vi "testRx.vi"() -> ()   [LabVIEW 2013]
uses:
  lv_lib/CHR34XXX.lvlib
panel:
  in  "通道号":u8 max=23 step=1
  out "devId":i32
  in  "Mode":u8
  in  "pstRsdcb":T1
  out "Exit":bool
  in  "退出":bool
  out "RxFlag":bool
  in  "开始接收":bool
  out "RxData(Hex)":string
  out "布尔":bool
  in  "通道号":u8 max=23 step=1
  # "Mode：通道模式，0 表示 232 模式，1 表示 422 模式，2 表示 485 模式 \nBaudRate：波特率\nRS232：75~500Kbps\nRS422/485：75~2.4Mbps\nByteSize：数据位长度，取值范围为 5~8\nStopBits：停止位个数，取值范围为 0~2\n取值为 0 时，表示 1 位停止位(ByteSize 取值为 5~8)\n取值为 1 时，表示 1.5 位停止位(ByteSize 取值为 5)\n取值为 2 时，表示 2 位停止位(ByteSize 取值为 6~8)\nParity：校验方式，取值范围为 0~4\n0：无校验，1：奇校验，2：偶校验，3：Mark 校验，4：Space 校验"
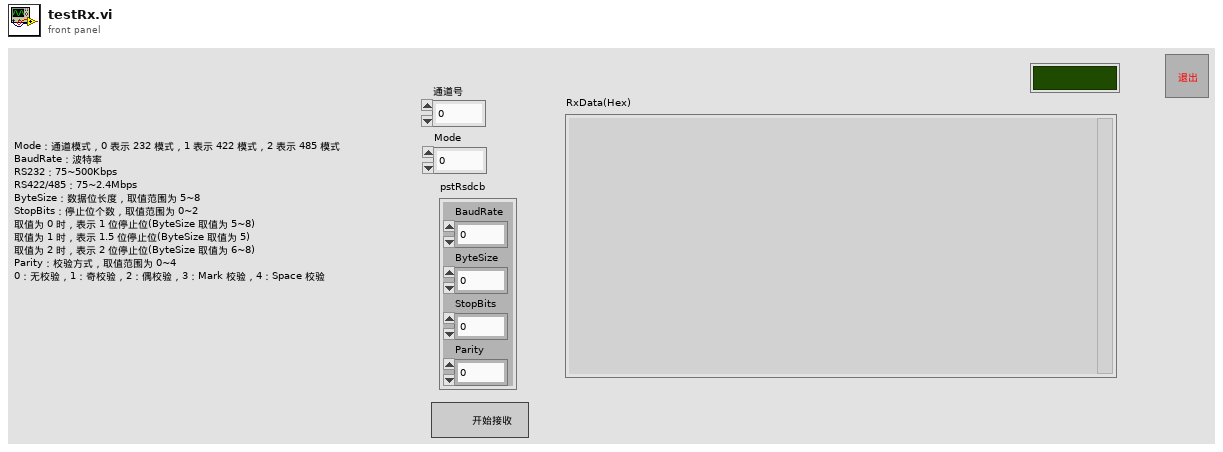
[diagram p1: front panel]
types:
  T1 = cluster{"BaudRate":u32, "ByteSize":u32, "StopBits":u32, "Parity":u32}
  T2 = enum8{"Enabled", "Disabled", "Disabled and Grayed Out"}
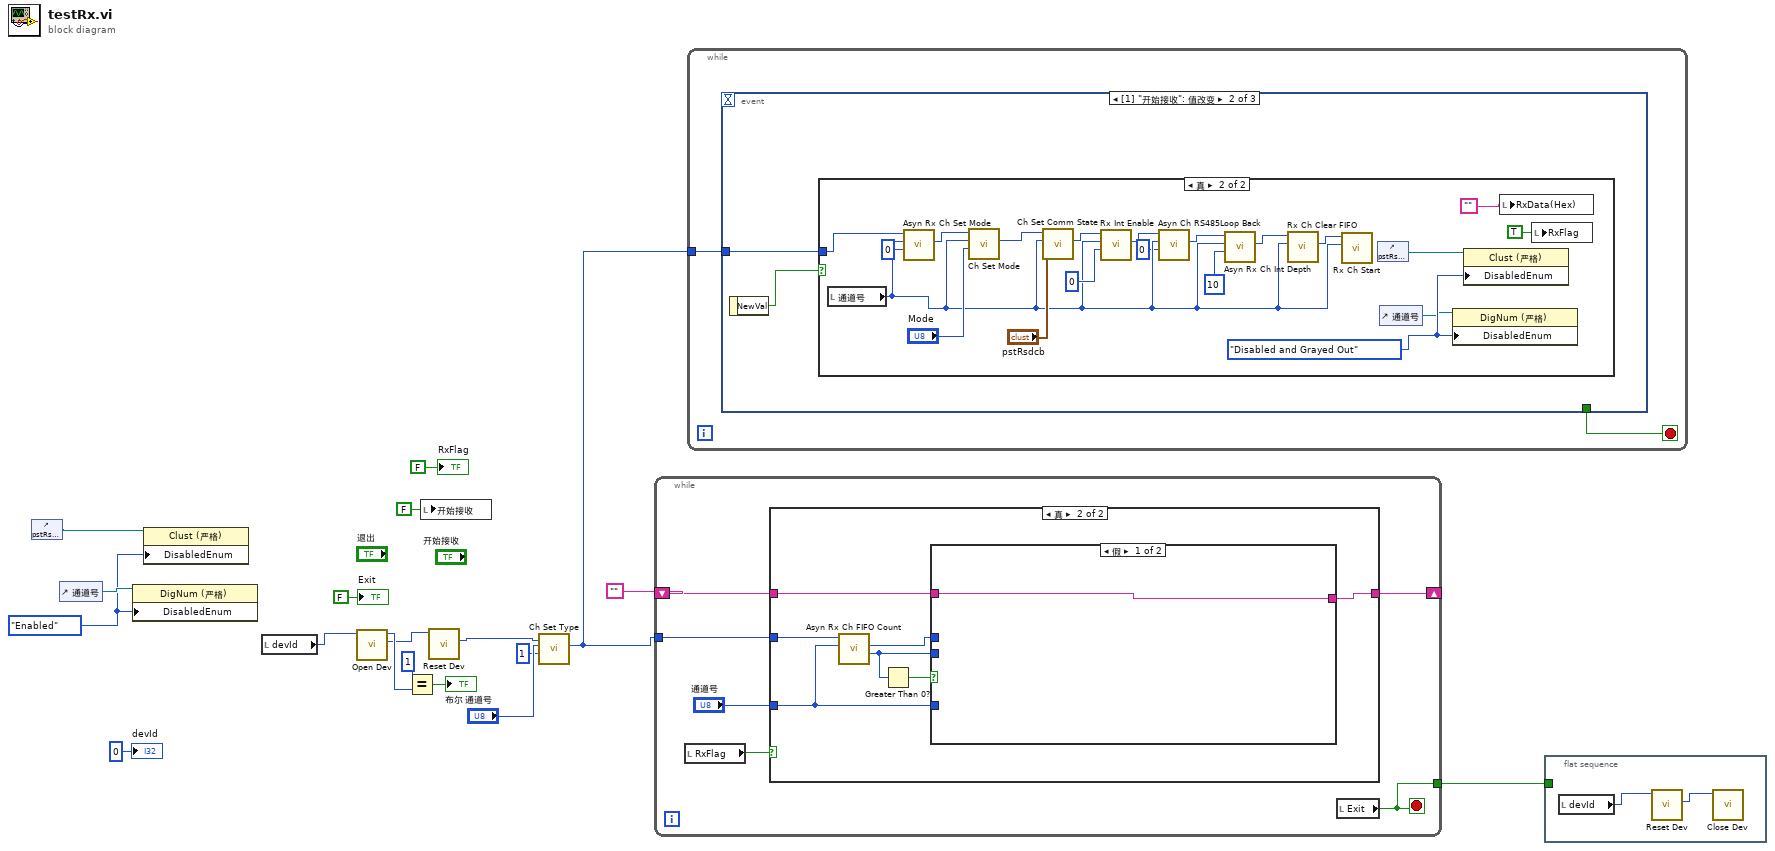
[diagram p0: block diagram]
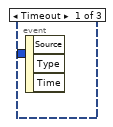
[diagram p2: hidden frame]
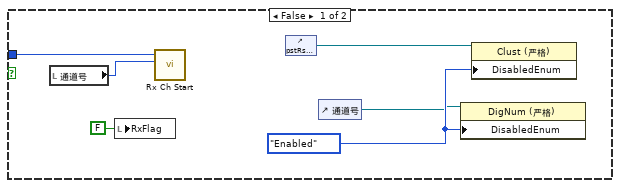
[diagram p3: hidden frame]
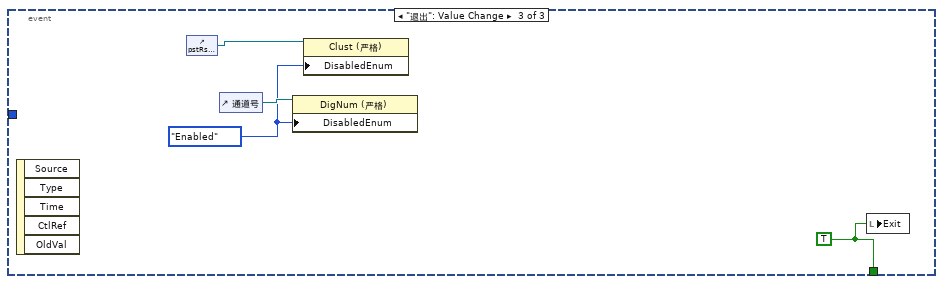
[diagram p4: hidden frame]
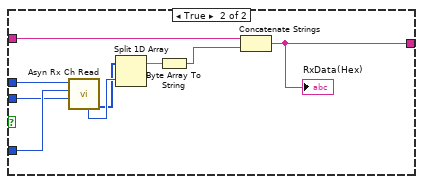
[diagram p6: hidden frame]
diagram:
  w10 = T2."Enabled" ("禁用")
  n1 = control-ref of="pstRsdcb"() -> (w9:refnum<vi>)
  n2 = control-ref of="通道号"() -> (w11:refnum<vi>)
  n3 = property class="DigNum (严格)"(reference=w11, "DisabledEnum"=w10) -> ()  [unwired: 1 in, 2 out]
  n4 = property class="Clust (严格)"(reference=w9, "DisabledEnum"=w10) -> ()  [unwired: 1 in, 2 out]
  n5 = local read "devId"() -> (w8:i32)
  n6 = call "Open Dev.vi"("devId in"=w8) -> ("devId out"=w2:i32, "function return"=w14:i32)  [unwired: 9 in]
  n7 = Equal?(x=1, y=w14) -> (x = y?=→"布尔":bool)
  n8 = local write "开始接收"(FALSE ("开始接收")) -> ()
  n9 = call "Reset Dev.vi"("devId"=w2) -> ("devId out"=w1:i32)  [unwired: 9 in, 1 out]
  n10 = call "Ch Set Type.vi"("Type"=u8 1, "Channel"="通道号", "devId"=w1) -> ("devId out"=w3:i32)  [unwired: 7 in, 1 out]
  n11 = while {
    tunnel: w3 -> [w24]
    shift-right: [w23] -> _
    shift-left: "" -> [w22]
    tunnel: [w19] -> w12
    stop <- w19 stop-if-true
    n12 = local read "RxFlag"() -> (w20:bool)
    n13 = case shown="真" w20 {
      tunnel: w24 -> [_ w32]
      tunnel: "通道号" -> [_ w30]
      tunnel: [w25 w28] -> w23
      tunnel: w22 -> [w25 w27]
      frame False {
      }
      frame True {
        n14 = call "Asyn Rx Ch FIFO Count.vi"("Channel"=w30, "devId"=w32) -> ("pCount out"=w29:u32, "devId out"=w26:i32)  [unwired: 7 in, 1 out]
        n15 = Greater Than 0?(x=w29) -> (x > 0?=w31:bool)
        n16 = case shown="假" w31 {
          tunnel: w26 -> [_ w42]
          tunnel: w30 -> [_ w41]
          tunnel: w29 -> [_ w40]
          tunnel: [w33 w35] -> w28
          tunnel: w27 -> [w33 w37]
          frame False {
          }
          frame True {
            n17 = call "Asyn Rx Ch Read.vi"("Length"=w40, "Channel"=w41, "devId"=w42) -> ("pBuffer out"=w34:u8[], "pReturned out"=w39:u32)  [unwired: 5 in, 2 out]
            n18 = Split 1D Array(array=w34, index=w39) -> (first subarray=w38:u8[])  [unwired: 1 out]
            n19 = Byte Array To String(unsigned byte array=w38) -> (string=w36:string)
            n20 = Concatenate Strings(w37, w36) -> (w35:string)
            "RxData(Hex)" <- w35
          }
        }
      }
    }
    n21 = local read "Exit"() -> (w19:bool)
  }
  n22 = while {
    tunnel: w3 -> [w44]
    stop <- w43 stop-if-true
    n23 = event shown="[1] \"开始接收\": 值改变" {
      selector: _ -> [_ _ _]
      dyn-events: _ -> [_ _ _]
      timeout: _ -> [_ _ _]
      tunnel: w44 -> [_ w46 _]
      tunnel: [_ _ w76] -> w43
      event Timeout {
        n24 = event-data() -> ()  [unwired: 1 in, 3 out]
      }
      event "开始接收": Value Change {
        n25 = event-data() -> ("NewVal"=w45:bool)  [unwired: 1 in]
        n26 = case shown="真" w45 {
          tunnel: w46 -> [w52 w61]
          frame False {
            w49 = T2."Enabled" ("禁用")
            n27 = local read "通道号"() -> (w51:u8)
            n28 = local write "RxFlag"(FALSE ("RxFlag")) -> ()
            n29 = call "Rx Ch Start.vi"("Channel"=w51, "devId"=w52) -> ()  [unwired: 8 in, 2 out]
            n30 = control-ref of="pstRsdcb"() -> (w47:refnum<vi>)
            n31 = control-ref of="通道号"() -> (w48:refnum<vi>)
            n32 = property class="DigNum (严格)"(reference=w48, "DisabledEnum"=w49) -> ()  [unwired: 1 in, 2 out]
            n33 = property class="Clust (严格)"(reference=w47, "DisabledEnum"=w49) -> ()  [unwired: 1 in, 2 out]
          }
          frame True {
            w69 = T2."Disabled and Grayed Out" ("禁用")
            n34 = local read "通道号"() -> (w54:u8)
            n35 = call "Asyn Rx Ch Set Mode.vi"("Mode"=u8 0, "Channel"=w54, "devId"=w61) -> ("devId out"=w59:i32)  [unwired: 7 in, 1 out]
            n36 = call "Ch Set Mode.vi"("Mode"="Mode", "Channel"=w54, "devId"=w59) -> ("devId out"=w67:i32)  [unwired: 7 in, 1 out]
            n37 = call "Ch Set Comm State.vi"("pstRsdcb"="pstRsdcb", "Channel"=w54, "devId"=w67) -> ("devId out"=w65:i32)  [unwired: 6 in, 2 out]
            n38 = call "Rx Int Enable.vi"("Enabled"=0, "Channel"=w54, "devId"=w65) -> ("devId out"=w55:i32)  [unwired: 7 in, 1 out]
            n39 = call "Asyn Ch RS485Loop Back.vi"("Enabled"=0, "Channel"=w54, "devId"=w55) -> ("devId out"=w58:i32)  [unwired: 7 in, 1 out]
            n40 = call "Asyn Rx Ch Int Depth.vi"("Depth"=10 ("Enabled"), "Channel"=w54, "devId"=w58) -> ("devId out"=w57:i32)  [unwired: 7 in, 1 out]
            n41 = call "Rx Ch Clear FIFO.vi"("Channel"=w54, "devId"=w57) -> ("devId out"=w56:i32)  [unwired: 8 in, 1 out]
            n42 = call "Rx Ch Start.vi"("Channel"=w54, "devId"=w56) -> ()  [unwired: 8 in, 2 out]
            n43 = control-ref of="pstRsdcb"() -> (w63:refnum<vi>)
            n44 = control-ref of="通道号"() -> (w68:refnum<vi>)
            n45 = property class="DigNum (严格)"(reference=w68, "DisabledEnum"=w69) -> ()  [unwired: 1 in, 2 out]
            n46 = property class="Clust (严格)"(reference=w63, "DisabledEnum"=w69) -> ()  [unwired: 1 in, 2 out]
            n47 = local write "RxData(Hex)"("") -> ()
            n48 = local write "RxFlag"(TRUE ("RxFlag")) -> ()
          }
        }
      }
      event "退出": Value Change {
        w74 = T2."Enabled" ("禁用")
        w76 = TRUE
        n49 = event-data() -> ()  [unwired: 1 in, 5 out]
        n50 = control-ref of="pstRsdcb"() -> (w73:refnum<vi>)
        n51 = control-ref of="通道号"() -> (w75:refnum<vi>)
        n52 = property class="DigNum (严格)"(reference=w75, "DisabledEnum"=w74) -> ()  [unwired: 1 in, 2 out]
        n53 = property class="Clust (严格)"(reference=w73, "DisabledEnum"=w74) -> ()  [unwired: 1 in, 2 out]
        n54 = local write "Exit"(w76) -> ()
      }
    }
  }
  n55 = flat-sequence {
    tunnel: w12 -> [_]
    frame #0 {
      n56 = local read "devId"() -> (w77:i32)
      n57 = call "Reset Dev.vi"("devId"=w77) -> ("devId out"=w78:i32)  [unwired: 9 in, 1 out]
      n58 = call "Close Dev.vi"("devId"=w78) -> ()  [unwired: 9 in, 2 out]
    }
  }
  "RxFlag" <- FALSE ("RxFlag")
  "Exit" <- FALSE ("Exit")
  "devId" <- 0 ("devId")
